vi "MSEditor_Script_SearchString.vi"(8 "error in (no error)":errorcluster, 9 "search string":refnum<vi>, 10 "Script of MS Process":refnum<vi>, 11 "search queue":refnum<queue>) -> (0 "error out":errorcluster)   [LabVIEW 2018]
uses:
  <vilib>/Utility/miscctls.llb/LVSelectionTypeDef.ctl
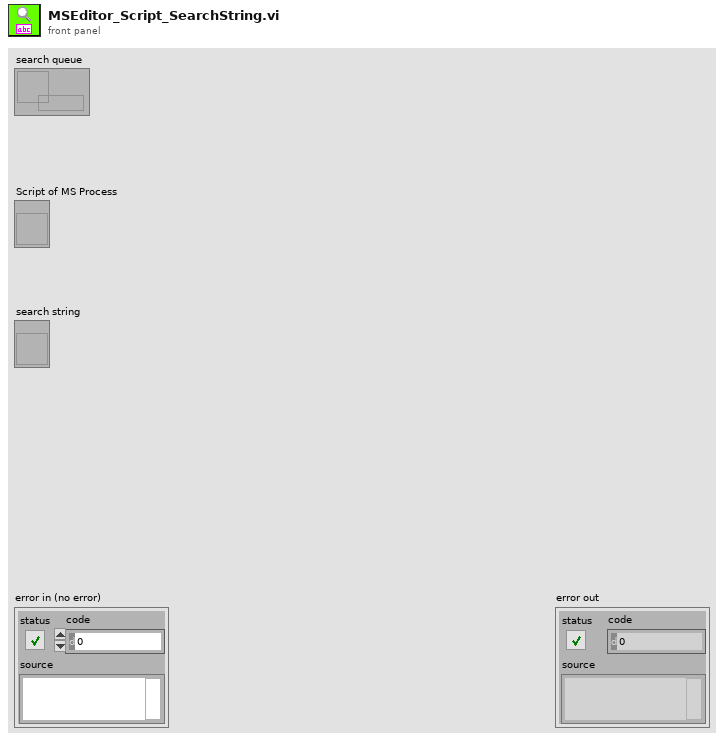
[diagram p1: front panel]
types:
  T1 = typedef "LVSelectionTypeDef.ctl" = cluster{"Selection Start":u32, "Selection End":u32}
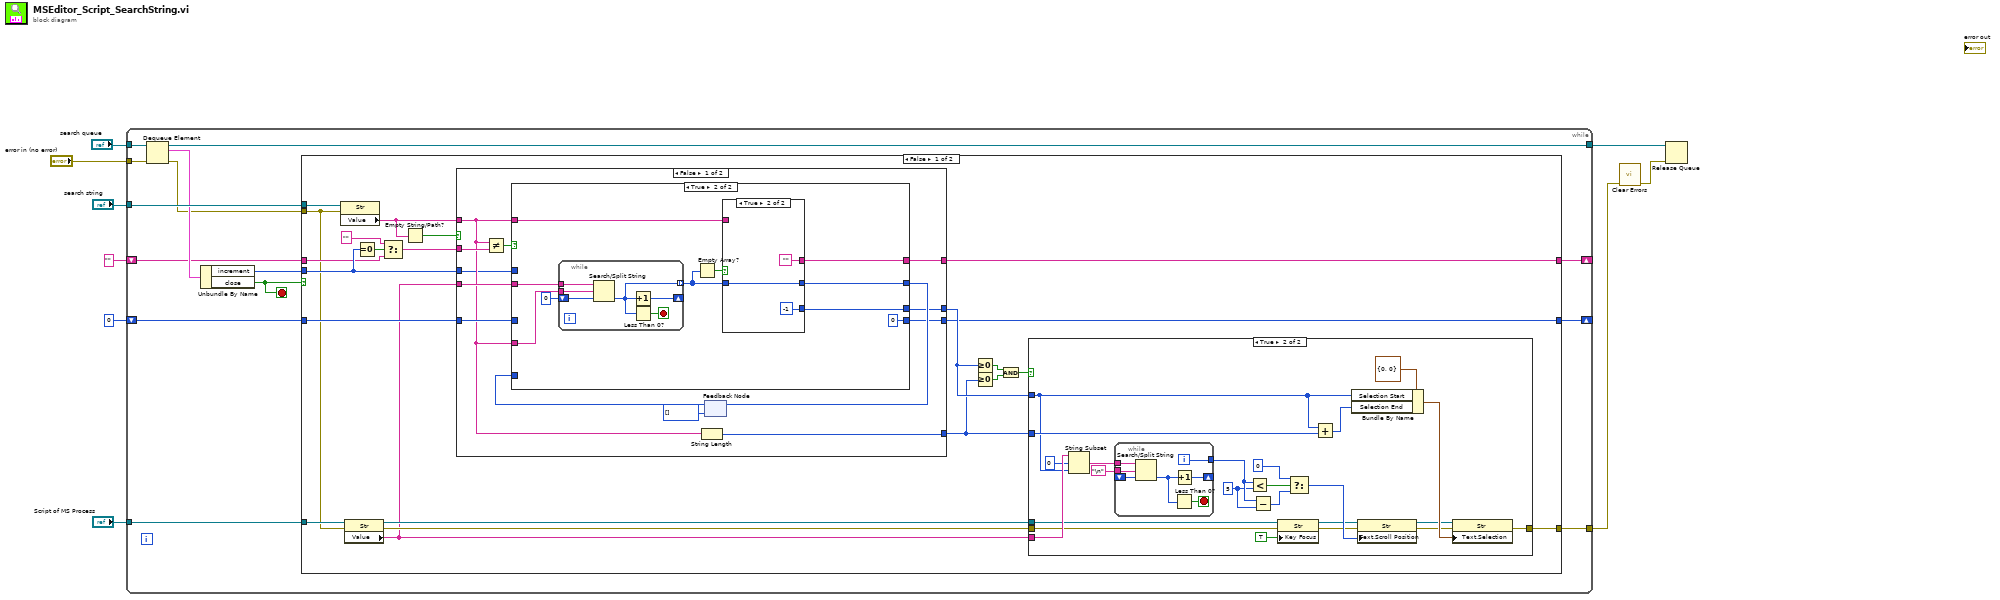
[diagram p0: block diagram]
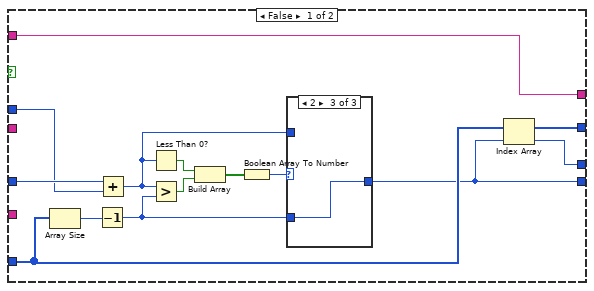
[diagram p3: hidden frame]
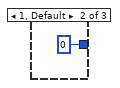
[diagram p5: hidden frame]
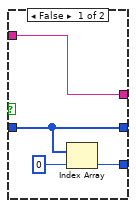
[diagram p6: hidden frame]
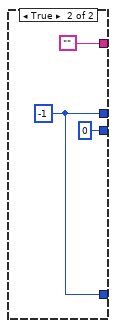
[diagram p7: hidden frame]
diagram:
  n1 = while {
    tunnel: "search string" -> [w23]
    tunnel: "Script of MS Process" -> [w21]
    shift-right: [w13] -> _
    shift-left: 0 -> [w19]
    shift-right: [w14] -> _
    shift-left: "" ("Value") -> [w15]
    tunnel: "error in (no error)" -> [w18]
    tunnel: "search queue" -> [w17]
    tunnel: [w11] -> w2
    tunnel: [w10] -> w3
    stop <- w12 stop-if-true
    n2 = Dequeue Element(queue=w17, error in (no error)=w18) -> (queue out=w11:refnum<queue>, element=w22:cluster{"increment":i32, "close":bool}, error out=w20:errorcluster)  [unwired: 1 in, 1 out]
    n3 = Unbundle By Name(w22) -> ("increment"=w16:i32, "close"=w12:bool)
    n4 = case shown="False" w12 {
      tunnel: w23 -> [w45 _]
      tunnel: w21 -> [w44 _]
      tunnel: w20 -> [w25 _]
      tunnel: w19 -> [w43 _]
      tunnel: w16 -> [w33 _]
      tunnel: w15 -> [w29 _]
      tunnel: [w27 _] -> w14
      tunnel: [w26 _] -> w13
      tunnel: [w24 _] -> w10
      frame False {
        n5 = property class="Str"(reference=w45, error in=w25) -> ("Value"=w42:string)  [unwired: 2 out]
        n6 = property class="Str"(reference=w44, error in=w25) -> (reference out=w35:refnum<vi>, error out=w34:errorcluster, "Value"=w28:string)
        n7 = Equal To 0?(x=w33) -> (x = 0?=w32:bool)
        n8 = Select(t="" ("Value"), s=w32, f=w29) -> (s? t:f=w30:string)
        n9 = Empty String/Path?(string/path=w42) -> (empty?=w41:bool)
        n10 = case shown="False" w41 {
          tunnel: w30 -> [w88 _]
          tunnel: w28 -> [w86 _]
          tunnel: w43 -> [w82 _]
          tunnel: [w81 0] -> w26
          tunnel: w42 -> [w80 _]
          tunnel: [w79 ""] -> w27
          tunnel: [w78 w128] -> w37
          tunnel: [w77 w128] -> w36
          tunnel: w33 -> [w76 _]
          frame False {
            n11 = Not Equal?(x=w80, y=w88) -> (x != y?=w87:bool)
            n12 = String Length(string=w80) -> (length=w77:i32)
            n13 = feedback #1(i32[] []) -> (w84:i32[])
            n14 = case shown="True" w87 {
              tunnel: [w99 w105] -> w85
              tunnel: w84 -> [w99 _]
              tunnel: w80 -> [_ w113]
              tunnel: w86 -> [_ w112]
              tunnel: [w101 w111] -> w78
              tunnel: w82 -> [w100 _]
              tunnel: [w93 0] -> w81
              tunnel: w80 -> [w92 w108]
              tunnel: [w92 w107] -> w79
              tunnel: w76 -> [w89 _]
              frame False {
                n15 = Array Size(array=w99) -> (size(s)=w91:i32)
                n16 = Decrement(x=w91) -> (x-1=w90:i32)
                n17 = Add(x=w100, y=w89) -> (x+y=w94:i32)
                n18 = Less Than 0?(x=w94) -> (x < 0?=w98:bool)
                n19 = Greater?(x=w94, y=w90) -> (0:w97:bool)
                n20 = Build Array(w98, w97) -> (w96:bool[])
                n21 = Boolean Array To Number(Boolean array=w96) -> (number=w95:u32)
                n22 = case shown="2" w95 {
                  tunnel: w94 -> [w102 _ _]
                  tunnel: w90 -> [_ _ w104]
                  tunnel: [w102 0 w104] -> w93
                  frame 0 {
                  }
                  frame 1, Default {
                  }
                  frame 2 {
                  }
                }
                n23 = Index Array(array=w99, index=w93) -> (element=w101:i32)
              }
              frame True {
                n24 = while {
                  tunnel: w112 -> [w127]
                  tunnel: w113 -> [w126]
                  tunnel: [w122] -> w106 mode=indexing
                  shift-right: [w123] -> _
                  shift-left: 0 -> [w125]
                  stop <- w124 stop-if-true
                  n25 = Search/Split String(string=w127, search string/char (-)=w126, offset (0)=w125) -> (offset of match=w122:i32)  [unwired: 2 out]
                  n26 = Increment(x=w122) -> (x+1=w123:i32)
                  n27 = Less Than 0?(x=w122) -> (x < 0?=w124:bool)
                }
                n28 = Empty Array?(array=w106) -> (empty?=w109:bool)
                n29 = case shown="True" w109 {
                  tunnel: [w117 -1 ("offset of match")] -> w111
                  tunnel: w106 -> [w115 w120]
                  tunnel: w108 -> [w116 _]
                  tunnel: [w116 ""] -> w107
                  tunnel: [w115 w120] -> w105
                  frame False {
                    n30 = Index Array(array=w115, index=0) -> (element=w117:i32)
                  }
                  frame True {
                  }
                }
              }
            }
            n31 = feedback-in #1(w85) -> ()
          }
          frame True {
            w128 = -1 ("offset of match")
          }
        }
        n32 = Greater Or Equal To 0?(x=w37) -> (x >= 0?=w40:bool)
        n33 = Greater Or Equal To 0?(x=w36) -> (x >= 0?=w39:bool)
        n34 = And(x=w40, y=w39) -> (x .and. y?=w38:bool)
        n35 = case shown="True" w38 {
          tunnel: w36 -> [_ w63]
          tunnel: w37 -> [_ w47]
          tunnel: w35 -> [_ w52]
          tunnel: w34 -> [_ w49]
          tunnel: w28 -> [_ w65]
          tunnel: [_ w46] -> w24
          frame False {
          }
          frame True {
            w58 = 5 ("y")
            n36 = String Subset(string=w65, offset (0)=0, length (rest)=w47) -> (substring=w62:string)
            n37 = while {
              tunnel: w62 -> [w75]
              tunnel: "\n" -> [w74]
              shift-right: [w71] -> _
              shift-left: _ -> [w73]
              tunnel: [w69] -> w59
              i -> [w69]
              stop <- w70 stop-if-true
              n38 = Search/Split String(string=w75, search string/char (-)=w74, offset (0)=w73) -> (offset of match=w72:i32)  [unwired: 2 out]
              n39 = Less Than 0?(x=w72) -> (x < 0?=w70:bool)
              n40 = Increment(x=w72) -> (x+1=w71:i32)
            }
            n41 = Less?(x=w59, y=w58) -> (x < y?=w61:bool)
            n42 = Subtract(x=w59, y=w58) -> (x-y=w57:i32)
            n43 = property class="Str"(reference=w52, error in=w49, "Key Focus"=TRUE) -> (reference out=w51:refnum<vi>, error out=w50:errorcluster)
            n44 = Select(t=0, s=w61, f=w57) -> (s? t:f=w56:i32)
            n45 = Add(x=w47, y=w63) -> (x+y=w68:i32)
            n46 = Bundle By Name(cluster=T1 {"Selection Start"=0, "Selection End"=0} ("Text.Selection"), "Selection Start"=w47, "Selection End"=w68) -> (w66:T1)
            n47 = property class="Str"(reference=w51, error in=w50, "Text.Scroll Position"=w56) -> (reference out=w55:refnum<vi>, error out=w54:errorcluster)
            n48 = property class="Str"(reference=w55, error in=w54, "Text.Selection"=w66) -> (error out=w46:errorcluster)  [unwired: 1 out]
          }
        }
      }
      frame True {
      }
    }
  }
  n49 = call <vilib>:"Clear Errors.vi"("error in (no error)"=w3) -> ("error out"=w1:errorcluster)  [unwired: 5 in, 1 out]
  n50 = Release Queue(queue=w2, error in (no error)=w1) -> ()  [unwired: 1 in, 3 out]
